vi "Configure Input.vi"(0 "VISA resource name":refnum<visa-resource-name>, 1 "Input Impedance (0: 50 ohms)":i32(ring) items=["50", "75"], 2 "External Frequency (0 Hz)":dbl, 5 "RF Calibrator (0: Off)":i32(ring) items=["Off", "50MHz", "4.8GHz", "COMB"], 9 "Input Coupling  (0: AC)":i32(ring) items=["AC", "DC"], 11 "error in (no error)":errorcluster, 12 "External Gain  (0 dB)":dbl, 13 "Frequency Reference In  (0:Sense)":i32(ring) items=["Sense", "Internal", "External"]) -> (4 "VISA resource name out":refnum<visa-resource-name>, 15 "error out":errorcluster)   [LabVIEW 2014, in "Agilent MXA Series.lvlib"]
doc: "Configures the input setting of the spectrum analyzer."
uses:
  Agilent MXA Series.lvlib
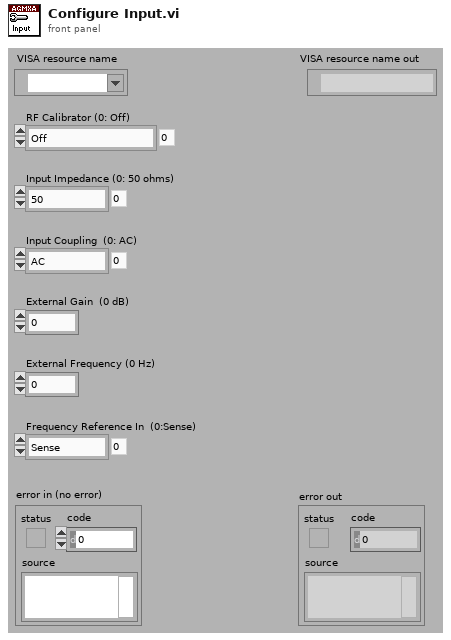
[diagram p1: front panel]
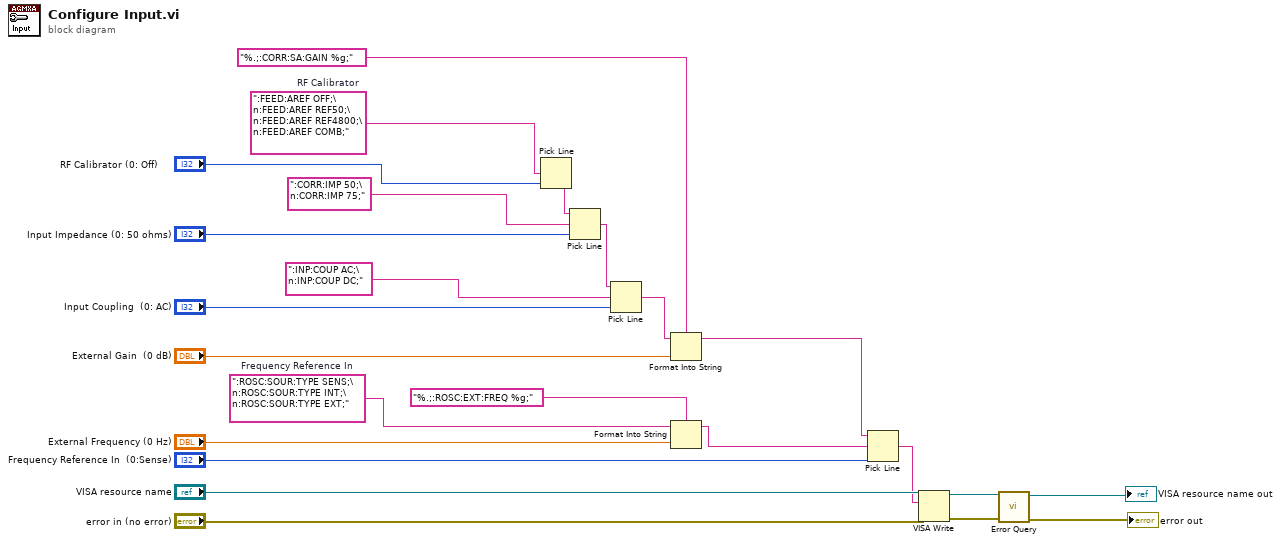
[diagram p0: block diagram]
diagram:
  w2 = ":ROSC:SOUR:TYPE SENS;\n:ROSC:SOUR:TYPE INT;\n:ROSC:SOUR:TYPE EXT;"  # Frequency Reference In
  w23 = ":FEED:AREF OFF;\n:FEED:AREF REF50;\n:FEED:AREF REF4800;\n:FEED:AREF COMB;"  # RF Calibrator
  n1 = Pick Line(multi-line string=w23, line index="RF Calibrator (0: Off)") -> (output string=w20:string)  [unwired: 1 in]
  n2 = Pick Line(string ("")=w20, multi-line string=":CORR:IMP 50;\n:CORR:IMP 75;", line index="Input Impedance (0: 50 ohms)") -> (output string=w17:string)
  n3 = Pick Line(string ("")=w17, multi-line string=":INP:COUP AC;\n:INP:COUP DC;", line index="Input Coupling  (0: AC)") -> (output string=w15:string)
  n4 = Format Into String(format string="%.;:CORR:SA:GAIN %g;", initial string=w15, "External Gain  (0 dB)") -> (resulting string=w10:string)  [unwired: 1 in, 1 out]
  n5 = Format Into String(format string="%.;:ROSC:EXT:FREQ %g;", initial string=w2, "External Frequency (0 Hz)") -> (resulting string=w1:string)  [unwired: 1 in, 1 out]
  n6 = Pick Line(string ("")=w10, multi-line string=w1, line index="Frequency Reference In  (0:Sense)") -> (output string=w3:string)
  n7 = VISA Write(VISA resource name="VISA resource name", write buffer=w3, error in (no error)="error in (no error)") -> (VISA resource name out=w6:refnum<visa-resource-name>, error out=w7:errorcluster)  [unwired: 1 out]
  n8 = call "Error Query.vi"("error in (no error)"=w7, "VISA resource name"=w6) -> ("error out"=→"error out":errorcluster, "VISA resource name out"=→"VISA resource name out":refnum<visa-resource-name>)  [unwired: 6 in, 2 out]
